vi "Init Handlers.vi"(8 "error in (no error)":errorcluster, 11 "Server in":refnum<class "Server.lvclass">) -> (0 "error out":errorcluster, 3 "Server out":refnum<class "Server.lvclass">)   [LabVIEW 2020, in "HTTP Server.lvlib" / "Server.lvclass"]
uses:
  Server.lvclass
  Server.lvclass/Server.ctl
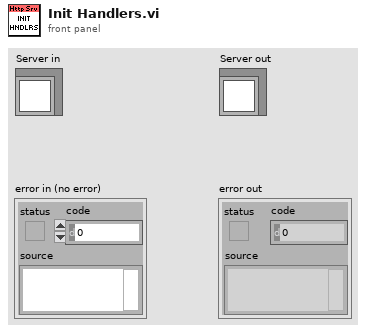
[diagram p1: front panel]
types:
  T1 = typedef "HTTP Server.lvlib/Server.lvclass/Ref Data.ctl" = cluster{"Connection Handler Map":T2, "Request Handler Map":T4, "Route Handler Map":T5, "Controller Handler Map":T6, "Controller Map":T7, "Response Handler Map":T8, "Complete Handler Map":T9, "Exception Handler Map":T10, "Connection Handler Index":u16, "Request Handler Index":u16, "Route Handler Index":u16, "Controller Handler Index":u16, "Controller Index":u16, "Response Handler Index":u16, "Complete Handler Index":u16, "Exception Handler Index":u16, "Services":refnum<class "Arguments.lvclass">}
  T2 = typedef "HTTP Server.lvlib/Connection Handler Map.ctl" = map{T3, refnum<class "Connection Handler.lvclass">}
  T3 = typedef "HTTP Server.lvlib/Priority.ctl" = cluster{"Entity":u16, "Index":u16}
  T4 = typedef "HTTP Server.lvlib/Request Handler Map.ctl" = map{T3, refnum<class "Request Handler.lvclass">}
  T5 = typedef "HTTP Server.lvlib/Route Handler Map.ctl" = map{T3, refnum<class "Route Handler.lvclass">}
  T6 = typedef "HTTP Server.lvlib/Controller Handler Map.ctl" = map{T3, refnum<class "Controller Handler.lvclass">}
  T7 = typedef "HTTP Server.lvlib/Controller Map.ctl" = map{T3, refnum<class "Controller.lvclass">}
  T8 = typedef "HTTP Server.lvlib/Response Handler Map.ctl" = map{T3, refnum<class "Response Handler.lvclass">}
  T9 = typedef "HTTP Server.lvlib/Complete Handler Map.ctl" = map{T3, refnum<class "Complete Handler.lvclass">}
  T10 = typedef "HTTP Server.lvlib/Exception Handler Map.ctl" = map{T3, refnum<class "Exception Handler.lvclass">}
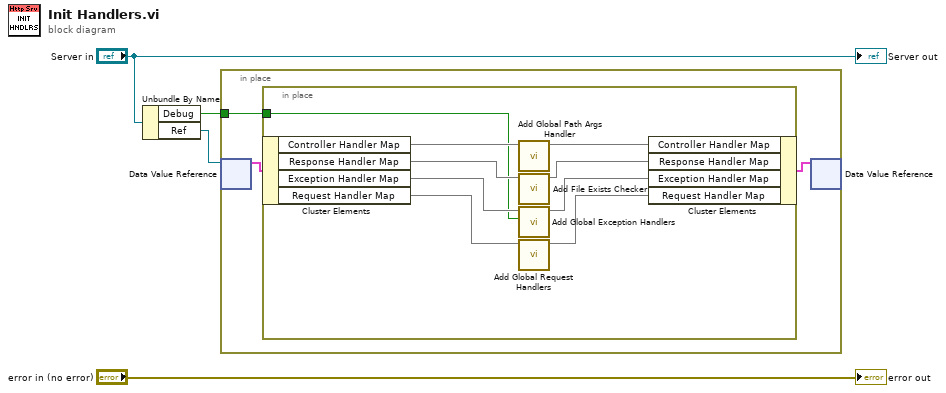
[diagram p0: block diagram]
diagram:
  n1 = Unbundle By Name("Server in") -> ("Debug"=w1:bool, "Ref"=w3:refnum<data-value>)
  n2 = in-place {
    in-place-border: w1 -> [w5]
    n3 = in-place-dvr #1(w3) -> (w7:T1)  [unwired: 1 out]
    n4 = in-place {
      in-place-border: w5 -> [w10]
      n5 = in-place-cluster #2(w7) -> ("Controller Handler Map"=w16:T6, "Response Handler Map"=w13:T8, "Exception Handler Map"=w12:T10, "Request Handler Map"=w9:T4)
      n6 = call "Add Global Path Args Handler.vi"("Controller Handler Map In"=w16) -> ("Controller Handler Map"=w15:T6)  [unwired: 10 in]
      n7 = call "Add File Exists Checker.vi"("Response Handler Map In"=w13) -> ("Response Handler Map"=w14:T8)  [unwired: 10 in]
      n8 = call "Add Global Exception Handlers.vi"("Debug"=w10, "Exception Handler Map In"=w12) -> ("Exception Handler Map"=w11:T10)  [unwired: 9 in]
      n9 = call "Add Global Request Handlers.vi"("Request Handler Map In"=w9) -> ("Request Handler Map"=w8:T4)  [unwired: 10 in]
      n10 = in-place-cluster #2("Controller Handler Map"=w15, "Response Handler Map"=w14, "Exception Handler Map"=w11, "Request Handler Map"=w8) -> (w6:T1)
    }
    n11 = in-place-dvr #1(w6) -> ()  [unwired: 2 out]
  }
  "error out" <- "error in (no error)"
  "Server out" <- "Server in"
